vi "Graphe 3D.vi"(4 "Nbre colonnes":i8=2 min=1, 5 "file path (dialog if empty)":path caption="chemin du fichier (boîte de dialogue si vide)", 6 "Paramètres axe Z":string[](array[string]), 7 "Nbre lignes entête":i8=2 min=1, 8 "N° colonne Y":i8=2 min=1, 9 "N° colonne X":i8=1 min=1) -> ()   [LabVIEW 2013]
uses:
  <vilib>/Platform/NI_3dgraph.lvlib
  <vilib>/Analysis/NI_AALBase.lvlib
panel:
  in  "Amplitudes":bool
  out "Go":bool
  in  "Init Vue":bool
  in  "Plan - Vue":i32(ring)=3 items=["Plan XY", "Plan XZ", "Plan YZ", "Vue 3D"]
  in  "System Link Text 4":bool
  in  "System Link Text 3":bool
  out "Ecart type":dbl caption="Ecart-type" format="%0.2f"
  in  "System Link Text 2":bool
  in  "System Link Text":bool
  out "Min":dbl
  out "Max":dbl
  out "Moyenne":dbl format="%0.2f"
  in  "Inverser échelle Y":bool caption="Inverser Y"
  in  "Inverser échelle x":bool caption="Inverser X"
  in  "Plot Style":i32(ring)=5 caption="Style de courbe" items=["Ligne"=1, "Point"=2, "Ligne - Point"=3, "Maillage"=4, "Surface"=5, "Surface - Ligne"=6, "Surface Normale"=7, "Contour Ligne"=8, "Surface Contour"=9]
  in  "Transparency (%)":dbl(slide) caption="Transparence (%)" scale=0.0..80.0
  in  "Quit":bool
  in  "Paramètre":u16(ring) items=["par", "TC01 dif", "TC20 dif"]
  in  "3D Surface 4":refnum<k7>(container) caption="Surface en 3D"
  in  "3D Surface 3":refnum<k7>(container) caption="Surface en 3D"
  in  "3D Surface 2":refnum<k7>(container) caption="Surface en 3D"
  in  "3D Surface":refnum<k7>(container) caption="Surface en 3D"
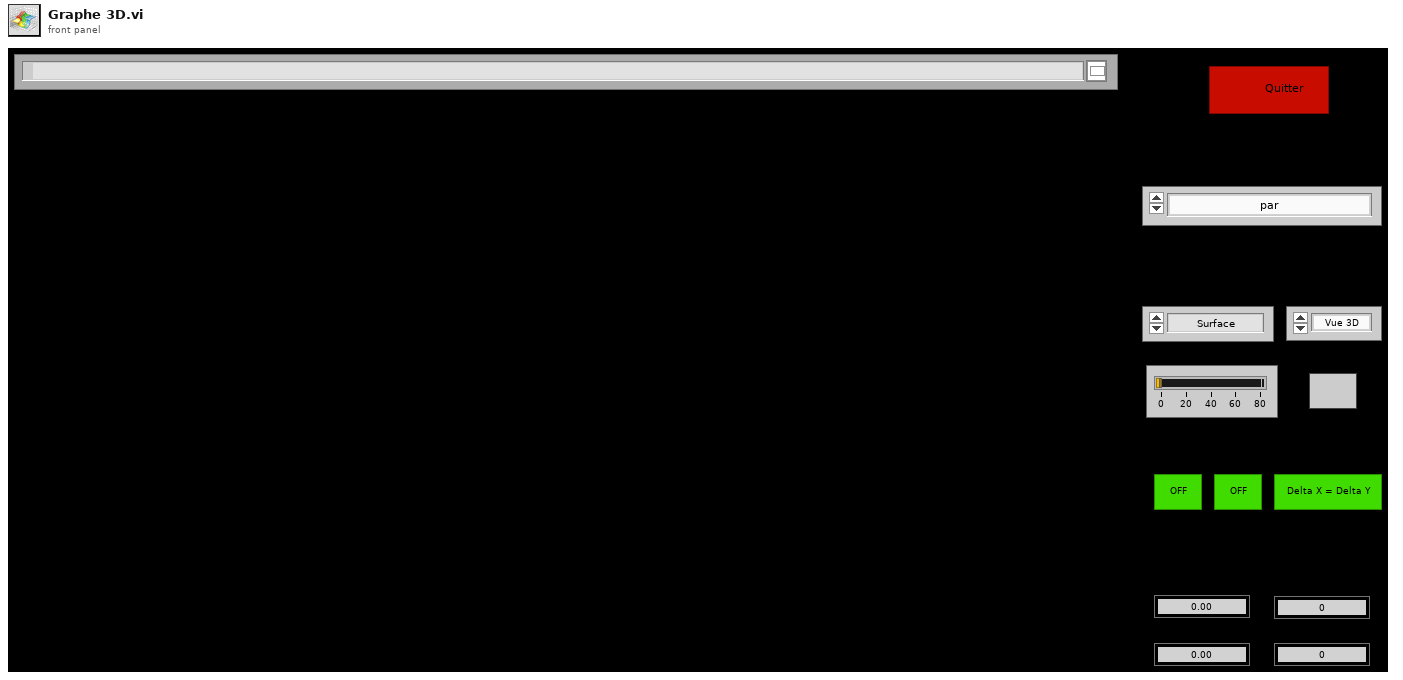
[diagram p1: front panel]
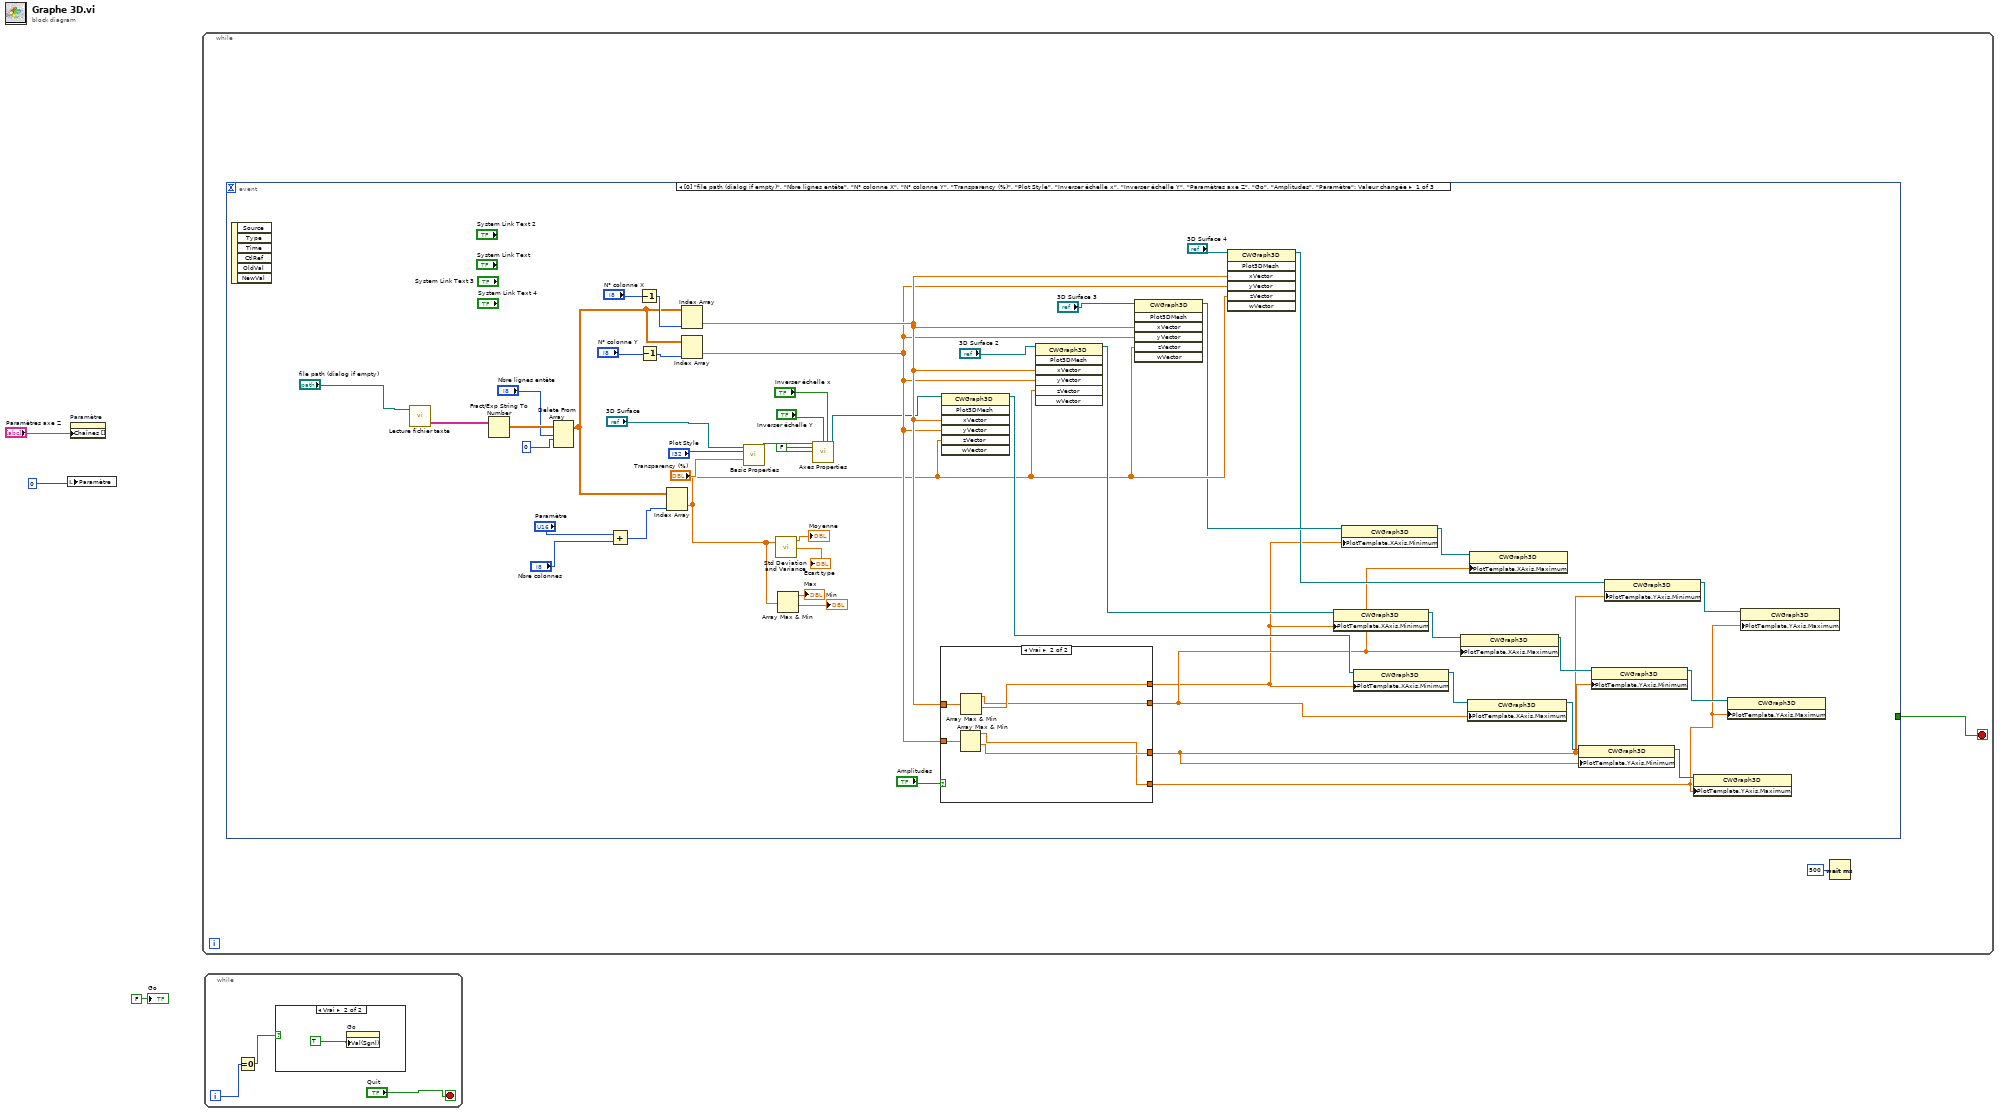
[diagram p0: block diagram]
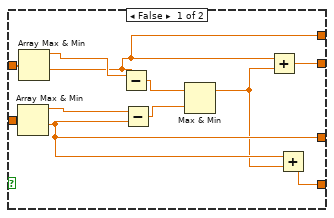
[diagram p3: hidden frame]
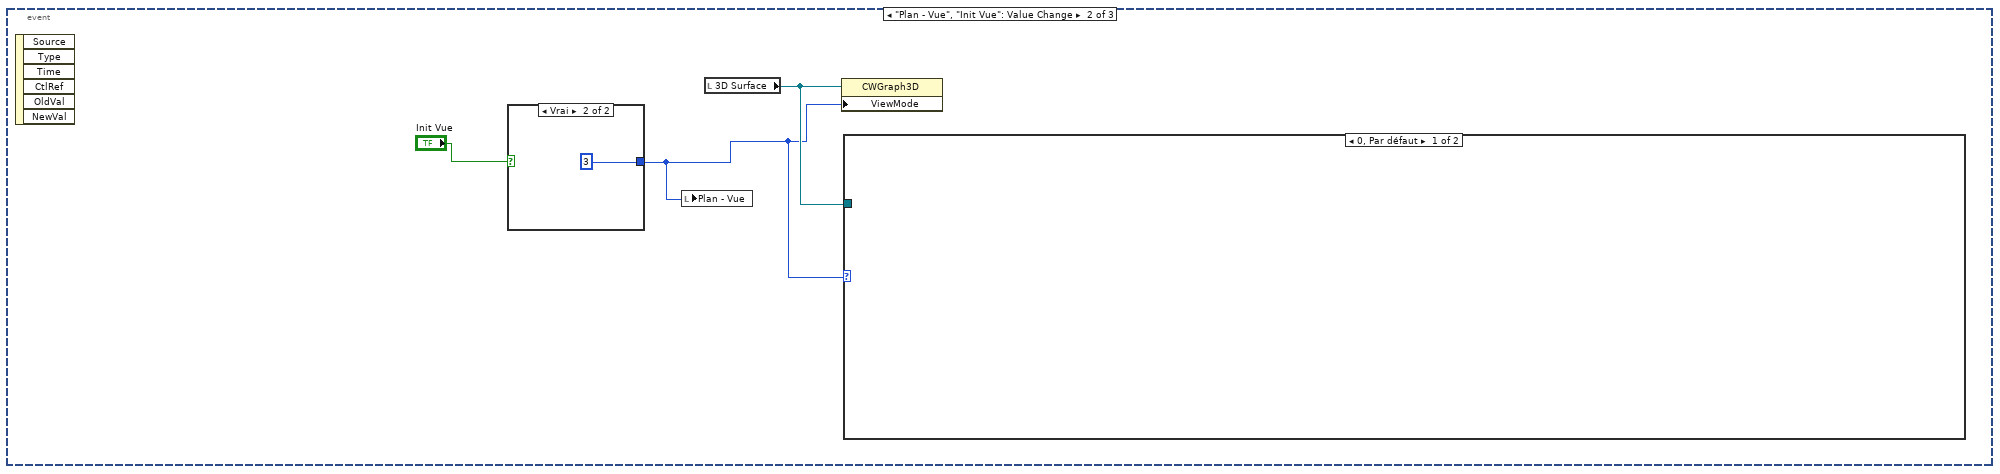
[diagram p4: hidden frame]
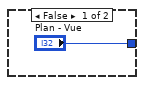
[diagram p5: hidden frame]
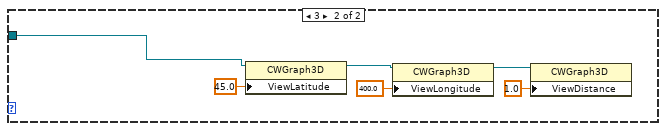
[diagram p6: hidden frame]
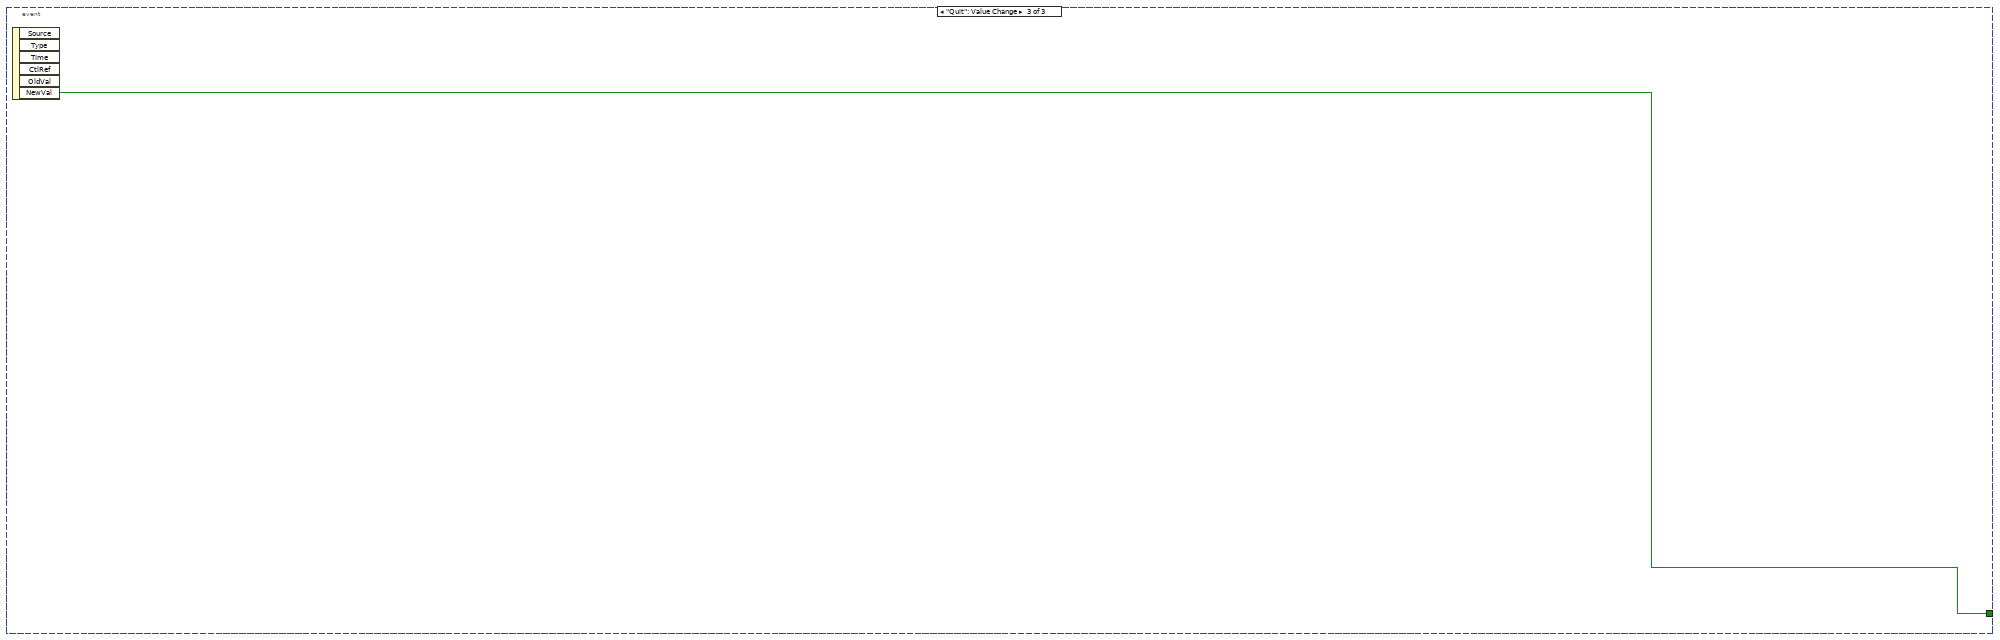
[diagram p7: hidden frame]
diagram:
  n1 = local write "Paramètre"(0) -> ()
  n2 = property on="Paramètre" class="MDér (strict)"("Chaînes []"="Paramètres axe Z") -> ()  [unwired: 2 in, 2 out]
  n3 = while {
    stop <- w4 stop-if-true
    n4 = event shown="[0] \"file path (dialog if empty)\", \"Nbre lignes entête\", \"N° colonne X\", \"N° colonne Y\", \"Transparency (%)\", \"Plot Style\", \"Inverser échelle x\", \"Inverser échelle Y\", \"Paramètres axe Z\", \"Go\", \"Amplitudes\", \"Paramètre\": Valeur changée" {
      selector: _ -> [_ _ _]
      dyn-events: _ -> [_ _ _]
      timeout: _ -> [_ _ _]
      tunnel: [_ _ w82] -> w4
      event "file path (dialog if empty)", "Nbre lignes entête", "N° colonne X", "N° colonne Y", "Transparency (%)", "Plot Style", "Inverser échelle x", "Inverser échelle Y", "Paramètres axe Z", "Go", "Amplitudes", "Paramètre": Value Change {
        w32 = FALSE ("auto scale x")
        n5 = event-data() -> ()  [unwired: 1 in, 6 out]
        n6 = call "Lecture fichier texte.vi"("file path (dialog if empty)"="file path (dialog if empty)") -> ("Table"=w52:string[][])  [unwired: 2 in, 1 out]
        n7 = Fract/Exp String To Number(string=w52) -> (number=w51:dbl[][])  [unwired: 3 in, 1 out]
        n8 = Delete From Array(array=w51, length="Nbre lignes entête", index (row)=0 ("indice (ligne)")) -> (array with subset deleted=w35:dbl[][])  [unwired: 1 in, 1 out]
        n9 = Add(x="Paramètre", y="Nbre colonnes") -> (x+y=w20:u16)
        n10 = Decrement(x="N° colonne X") -> (x-1=w46:i8)
        n11 = Decrement(x="N° colonne Y") -> (x-1=w48:i8)
        n12 = Index Array(array=w35, index (col)=w20) -> (element=w27:dbl[])  [unwired: 1 in]
        n13 = Index Array(array=w35, index (col)=w46) -> (element=w34:dbl[])  [unwired: 1 in]
        n14 = Index Array(array=w35, index (col)=w48) -> (element=w33:dbl[])  [unwired: 1 in]
        n15 = call <vilib>:"Basic Properties.vi"("3D graph"="3D Surface", "plot style"="Plot Style", "transparency"="Transparency (%)") -> ("3D graph out"=w45:refnum<k7>)  [unwired: 11 in, 1 out]
        n16 = call <vilib>:"Std Deviation and Variance.vi"("X"=w27) -> ("mean"=→"Moyenne":dbl, "standard deviation"=→"Ecart type":dbl)  [unwired: 1 in, 1 out]
        n17 = Array Max & Min(array=w27) -> (max value=→"Max":dbl, min value=→"Min":dbl)  [unwired: 2 out]
        n18 = call <vilib>:"Axes Properties.vi"("3D graph"=w45, "invert y"="Inverser échelle Y", "invert x"="Inverser échelle x", "auto scale x"=w32, "auto scale y"=w32) -> ("3D graph out"=w31:refnum<k7>)  [unwired: 9 in, 1 out]
        n19 = case shown="Vrai" "Amplitudes" {
          tunnel: w34 -> [w64 w70]
          tunnel: w33 -> [w63 w69]
          tunnel: [w60 w65] -> w10
          tunnel: [w59 w66] -> w9
          tunnel: [w58 w67] -> w8
          tunnel: [w57 w68] -> w7
          frame False {
            n20 = Array Max & Min(array=w63) -> (max value=w61:dbl, min value=w59:dbl)  [unwired: 2 out]
            n21 = Array Max & Min(array=w64) -> (max value=w62:dbl, min value=w57:dbl)  [unwired: 2 out]
            n22 = Subtract(x=w62, y=w57) -> (x-y=w56:dbl)
            n23 = Subtract(x=w61, y=w59) -> (x-y=w55:dbl)
            n24 = Max & Min(x=w56, y=w55) -> (max(x,y)=w54:dbl)  [unwired: 1 out]
            n25 = Add(x=w57, y=w54) -> (x+y=w58:dbl)
            n26 = Add(x=w59, y=w54) -> (x+y=w60:dbl)
          }
          frame True {
            n27 = Array Max & Min(array=w69) -> (max value=w65:dbl, min value=w66:dbl)  [unwired: 2 out]
            n28 = Array Max & Min(array=w70) -> (max value=w67:dbl, min value=w68:dbl)  [unwired: 2 out]
          }
        }
        n29 = invoke class="CWGraph3D" method="Plot3DMesh"(reference=w31, "xVector"=w34, "yVector"=w33, "zVector"=w27) -> (reference out=w30:refnum<k7>)  [unwired: 3 in, 6 out]
        n30 = invoke class="CWGraph3D" method="Plot3DMesh"(reference="3D Surface 2", "xVector"=w34, "yVector"=w33, "zVector"=w27) -> (reference out=w28:refnum<k7>)  [unwired: 3 in, 6 out]
        n31 = invoke class="CWGraph3D" method="Plot3DMesh"(reference="3D Surface 3", "xVector"=w34, "yVector"=w33, "zVector"=w27) -> (reference out=w24:refnum<k7>)  [unwired: 3 in, 6 out]
        n32 = invoke class="CWGraph3D" method="Plot3DMesh"(reference="3D Surface 4", "xVector"=w34, "yVector"=w33, "zVector"=w27) -> (reference out=w23:refnum<k7>)  [unwired: 3 in, 6 out]
        n33 = property class="CWGraph3D"(reference=w28, "PlotTemplate.XAxis.Minimum"=w7) -> (reference out=w15:refnum<k7>)  [unwired: 1 in, 1 out]
        n34 = property class="CWGraph3D"(reference=w24, "PlotTemplate.XAxis.Minimum"=w7) -> (reference out=w12:refnum<k7>)  [unwired: 1 in, 1 out]
        n35 = property class="CWGraph3D"(reference=w30, "PlotTemplate.XAxis.Minimum"=w7) -> (reference out=w18:refnum<k7>)  [unwired: 1 in, 1 out]
        n36 = property class="CWGraph3D"(reference=w15, "PlotTemplate.XAxis.Maximum"=w8) -> (reference out=w14:refnum<k7>)  [unwired: 1 in, 1 out]
        n37 = property class="CWGraph3D"(reference=w18, "PlotTemplate.XAxis.Maximum"=w8) -> (reference out=w16:refnum<k7>)  [unwired: 1 in, 1 out]
        n38 = property class="CWGraph3D"(reference=w12, "PlotTemplate.XAxis.Maximum"=w8) -> ()  [unwired: 1 in, 2 out]
        n39 = property class="CWGraph3D"(reference=w16, "PlotTemplate.YAxis.Minimum"=w9) -> (reference out=w17:refnum<k7>)  [unwired: 1 in, 1 out]
        n40 = property class="CWGraph3D"(reference=w14, "PlotTemplate.YAxis.Minimum"=w9) -> (reference out=w13:refnum<k7>)  [unwired: 1 in, 1 out]
        n41 = property class="CWGraph3D"(reference=w23, "PlotTemplate.YAxis.Minimum"=w9) -> (reference out=w11:refnum<k7>)  [unwired: 1 in, 1 out]
        n42 = property class="CWGraph3D"(reference=w17, "PlotTemplate.YAxis.Maximum"=w10) -> ()  [unwired: 1 in, 2 out]
        n43 = property class="CWGraph3D"(reference=w13, "PlotTemplate.YAxis.Maximum"=w10) -> ()  [unwired: 1 in, 2 out]
        n44 = property class="CWGraph3D"(reference=w11, "PlotTemplate.YAxis.Maximum"=w10) -> ()  [unwired: 1 in, 2 out]
      }
      event "Plan - Vue", "Init Vue": Value Change {
        n45 = event-data() -> ()  [unwired: 1 in, 6 out]
        n46 = case shown="Vrai" "Init Vue" {
          tunnel: ["Plan - Vue" 3 ("Plan - Vue")] -> w71
          frame False {
          }
          frame True {
          }
        }
        n47 = local write "Plan - Vue"(w71) -> ()
        n48 = local read "3D Surface"() -> (w73:refnum<k7>)
        n49 = property class="CWGraph3D"(reference=w73, "ViewMode"=w71) -> ()  [unwired: 1 in, 2 out]
        n50 = case shown="0, Par défaut" w71 {
          tunnel: w73 -> [_ w76]
          frame 0, Default {
          }
          frame 3 {
            n51 = property class="CWGraph3D"(reference=w76, "ViewLatitude"=45.0) -> (reference out=w79:refnum<k7>)  [unwired: 1 in, 1 out]
            n52 = property class="CWGraph3D"(reference=w79, "ViewLongitude"=400.0) -> (reference out=w81:refnum<k7>)  [unwired: 1 in, 1 out]
            n53 = property class="CWGraph3D"(reference=w81, "ViewDistance"=1.0) -> ()  [unwired: 1 in, 2 out]
          }
        }
      }
      event "Quit": Value Change {
        n54 = event-data() -> ("NewVal"=w82:bool)  [unwired: 1 in, 5 out]
      }
    }
    n55 = Wait (ms)(milliseconds to wait=u32 500 ("attente (ms)")) -> ()  [unwired: 1 out]
  }
  n56 = while {
    i -> [w84]
    stop <- "Quit" stop-if-true
    n57 = Equal To 0?(x=w84) -> (x = 0?=w85:bool)
    n58 = case shown="Vrai" w85 {
      frame False {
      }
      frame True {
        n59 = property on="Go" class="Bool"("Val(Sgnl)"=TRUE) -> ()  [unwired: 2 in, 2 out]
      }
    }
  }
  "Go" <- FALSE ("Go")
